vi "Place_CFD_cursors.vi"(9 "CFD in":i32, 10 "CFD 3":i32, 11 "WaveformGraph in":refnum<vi>) -> (3 "CFD out":dbl)   [LabVIEW 2019]
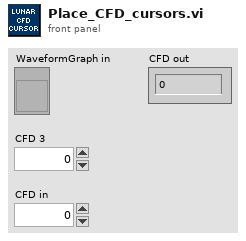
[diagram p1: front panel]
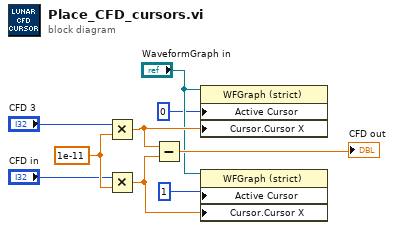
[diagram p0: block diagram]
diagram:
  w3 = 1e-11
  n1 = Multiply(x="CFD 3", y=w3) -> (x*y=w7:dbl)
  n2 = Multiply(x="CFD in", y=w3) -> (x*y=w8:dbl)
  n3 = Subtract(x=w7, y=w8) -> (x-y=→"CFD out":dbl)
  n4 = property on="Property Node" class="WFGraph (strict)"(reference="WaveformGraph in", "Active Cursor"=u32 0, "Cursor.Cursor X"=w7) -> ()  [unwired: 1 in, 2 out]
  n5 = property on="Property Node" class="WFGraph (strict)"(reference="WaveformGraph in", "Active Cursor"=u32 1, "Cursor.Cursor X"=w8) -> ()  [unwired: 1 in, 2 out]
